vi "Motor_Limit.vi"(0 "Current_Pos":dbl, 1 "Motor_Speed":dbl, 2 "Forward_StartScale":dbl, 3 "Reverse_StartScale":dbl, 4 "Forward_Limit":dbl, 5 "Reverse_Limit":dbl) -> (14 "New_Motor_Speed":dbl)   [LabVIEW 2016]
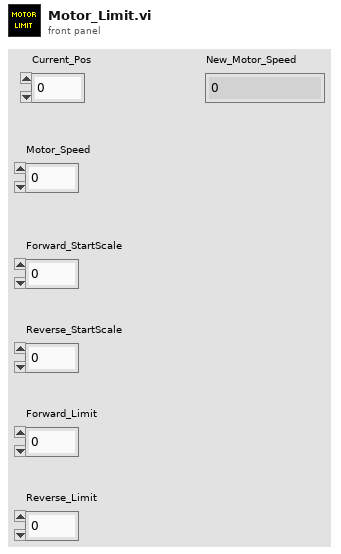
[diagram p1: front panel]
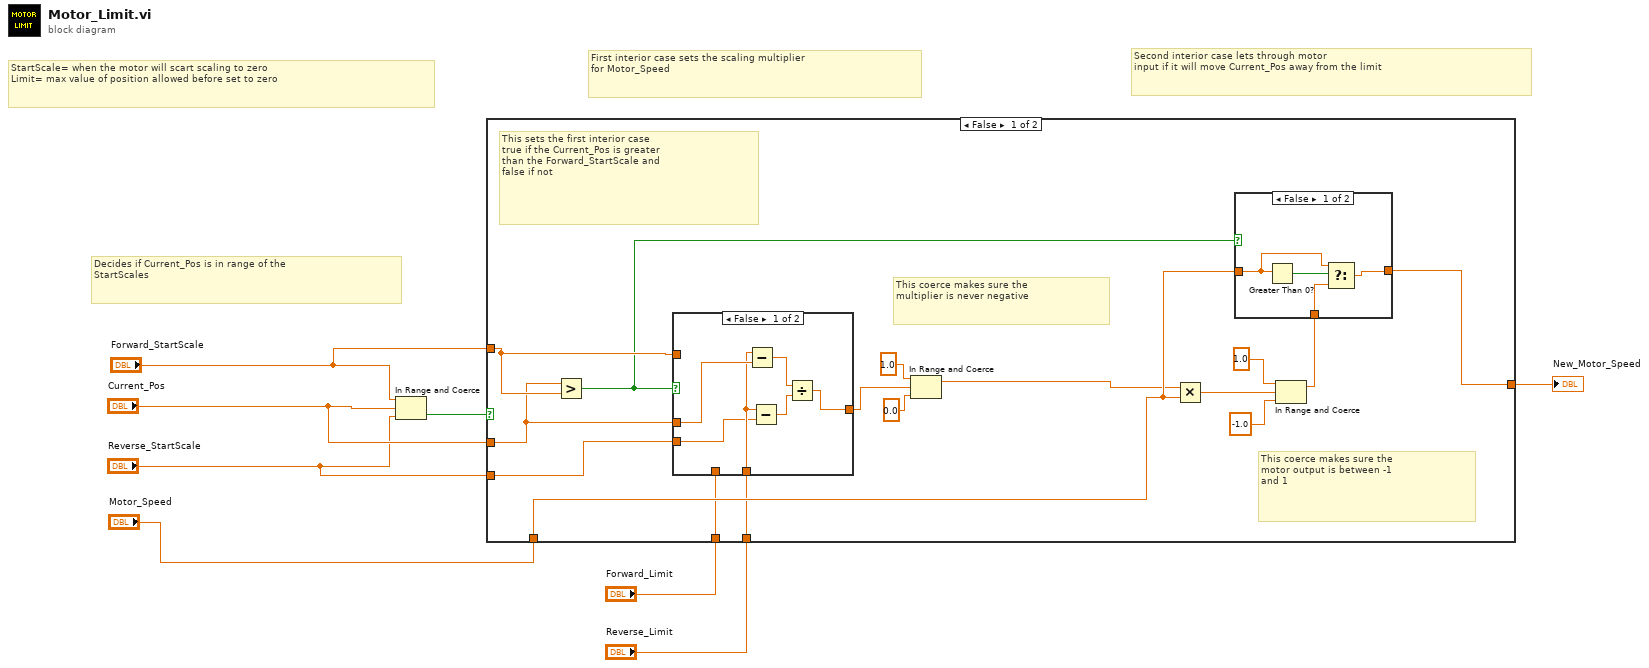
[diagram p0: block diagram]
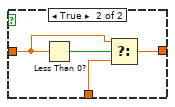
[diagram p2: hidden frame]
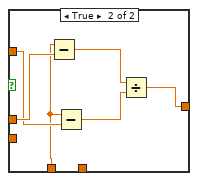
[diagram p3: hidden frame]
diagram:
  # "Second interior case lets through motor \ninput if it will move Current_Pos away from the limit"
  # "First interior case sets the scaling multiplier\nfor Motor_Speed"
  # "Decides if Current_Pos is in range of the\nStartScales"
  # "StartScale= when the motor will scart scaling to zero\nLimit= max value of position allowed before set to zero"
  n1 = In Range and Coerce(upper limit="Forward_StartScale", x="Current_Pos", lower limit="Reverse_StartScale") -> (In Range?=w8:bool)  [unwired: 1 out]
  n2 = case shown="False" w8 {
    tunnel: "Motor_Speed" -> [w18 w45]
    tunnel: [w9 w45] -> w6
    tunnel: "Current_Pos" -> [w16 _]
    tunnel: "Forward_StartScale" -> [w23 _]
    tunnel: "Reverse_StartScale" -> [w24 _]
    tunnel: "Forward_Limit" -> [w14 _]
    tunnel: "Reverse_Limit" -> [w15 _]
    frame False {
      # "This coerce makes sure the \nmotor output is between -1\nand 1"
      # "This coerce makes sure the\nmultiplier is never negative"
      # "This sets the first interior case\ntrue if the Current_Pos is greater \nthan the Forward_StartScale and\nfalse if not"
      n3 = Greater?(x=w16, y=w23) -> (0:w19:bool)
      n4 = case shown="False" w19 {
        tunnel: w24 -> [w33 _]
        tunnel: w23 -> [_ w43]
        tunnel: w16 -> [w37 w44]
        tunnel: w14 -> [_ w42]
        tunnel: w15 -> [w34 _]
        tunnel: [w38 w39] -> w13
        frame False {
          n5 = Subtract(x=w34, y=w37) -> (x-y=w36:dbl)
          n6 = Subtract(x=w34, y=w33) -> (x-y=w35:dbl)
          n7 = Divide(x=w36, y=w35) -> (x/y=w38:dbl)
        }
        frame True {
          n8 = Subtract(x=w42, y=w44) -> (x-y=w41:dbl)
          n9 = Subtract(x=w42, y=w43) -> (x-y=w40:dbl)
          n10 = Divide(x=w41, y=w40) -> (x/y=w39:dbl)
        }
      }
      n11 = In Range and Coerce(upper limit=1.0, x=w13, lower limit=0.0) -> (coerced(x)=w10:dbl)  [unwired: 1 out]
      n12 = Multiply(x=w10, y=w18) -> (x*y=w20:dbl)
      n13 = In Range and Coerce(upper limit=1.0, x=w20, lower limit=-1.0) -> (coerced(x)=w17:dbl)  [unwired: 1 out]
      n14 = case shown="False" w19 {
        tunnel: w18 -> [w25 w31]
        tunnel: w17 -> [w26 w30]
        tunnel: [w28 w29] -> w9
        frame False {
          n15 = Greater Than 0?(x=w25) -> (x > 0?=w27:bool)
          n16 = Select(t=w25, s=w27, f=w26) -> (s? t:f=w28:dbl)
        }
        frame True {
          n17 = Less Than 0?(x=w31) -> (x < 0?=w32:bool)
          n18 = Select(t=w31, s=w32, f=w30) -> (s? t:f=w29:dbl)
        }
      }
    }
    frame True {
      # "Passes through Motor_Speed if \nCurrent_Pos is in range"
    }
  }
  "New_Motor_Speed" <- w6
